vi "UpdateWindowSurfaceRects.vi"(8 "No Error":errorcluster, 10 "Rects":T1[](array[typedef]), 11 "Window [SDL_Window *]":T2 format="%.0x") -> (0 "Error Out":errorcluster)   [LabVIEW 2026, in "SDL3.lvlib" / "Video.lvlib"]
doc: "<B>Summary</B>\nCopy areas of the window surface to the screen.\n\n<B>Remarks</B>\nThis is the function you use to reflect changes to portions of the surface on the screen.\n\nThis function is equivalent to the SDL 1.2 API <B>SDL_UpdateRects()</B>.\n\nNote that this function will update at least the rectangles specified, but this is only intended as an optimization; in practice, this might update more of the screen (or all of the screen!), depending on what method SDL uses to send pixels to the system."
uses:
  Video.lvlib
  Rect/Rect--cluster.ctl
  <vilib>/Utility/error.llb/Error Cluster From Error Code.vi
  Error/Error.lvlib
  Lib/SDL3.dll
  Rect/Rect.lvlib
  SDL_Window--pointer.ctl
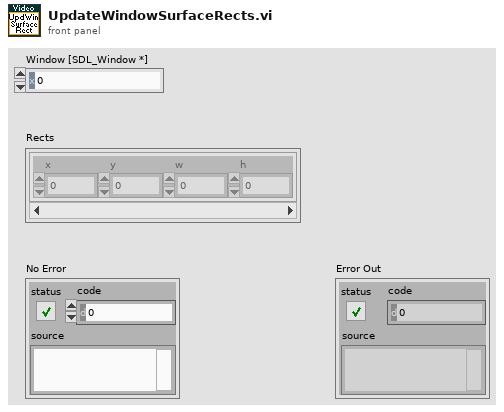
[diagram p1: front panel]
types:
  T1 = typedef "SDL3.lvlib/Rect.lvlib/Rect--cluster.ctl" = cluster{"x":i32, "y":i32, "w":i32, "h":i32}
  T2 = typedef "SDL3.lvlib/Video.lvlib/SDL_Window--pointer.ctl" = i64
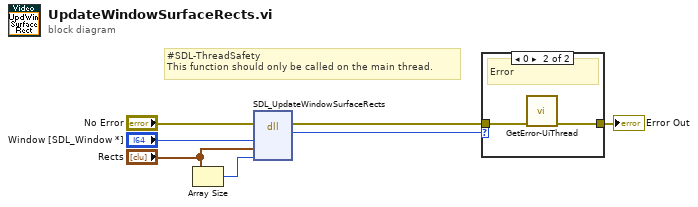
[diagram p0: block diagram]
diagram:
  # "#SDL-ThreadSafety\nThis function should only be called on the main thread."
  n1 = Array Size(array="Rects") -> (size(s)=w2:i32)
  n2 = dll-call lib="C:/Users/saukko/Dev/LV-SDL3/Sources/SDL3/Lib/SDL3.*" fn="SDL_UpdateWindowSurfaceRects"(error in="No Error", "window"="Window [SDL_Window *]", "rects"="Rects", "numrects"=w2) -> (error out=w5:errorcluster, "return type"=w3:i32)  [unwired: 5 in, 1 out]
  n3 = case shown="0" w3 {
    tunnel: w5 -> [w8 w10]
    tunnel: [w8 w9] -> w4
    frame Default {
      # "Ok"
    }
    frame 0 {
      # "Error"
      n4 = call "GetError-UiThread.vi"("No Error"=w10) -> ("error out"=w9:errorcluster)  [unwired: 10 in]
    }
  }
  "Error Out" <- w4
